vi "Pseudo_RNG.vi"() -> (3 "pseudo random value":u16)   [LabVIEW 2018]
doc: "This VI generates a sequence of pseudo random numbers using a linear feedback shift register algorithm with four taps.\n\nhttp://en.wikipedia.org/wiki/Linear_feedback_shift_register"
uses:
  <vilib>/rvi/Emulation/niFpgaSctlEmulationGetInTimedLoop.vi
  <vilib>/rvi/Emulation/niFpgaProcessEmulError.vi
  Instance           1 45Saved   Pseudo Random Number Generator (FPGA) .vi
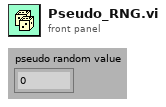
[diagram p1: front panel]
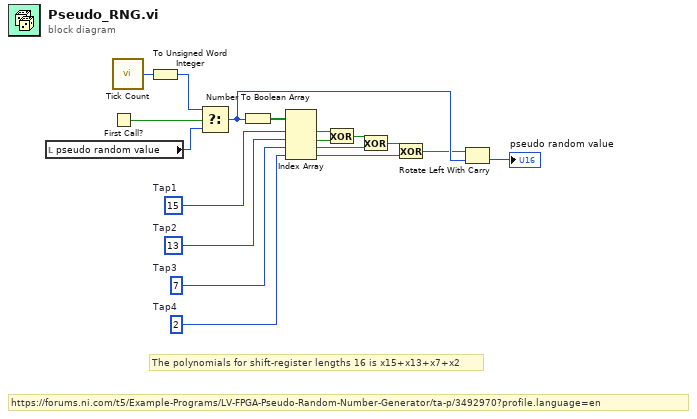
[diagram p0: block diagram]
diagram:
  w10 = 2  # Tap4
  w11 = 7  # Tap3
  w16 = 13  # Tap2
  w17 = 15  # Tap1
  # "https://forums.ni.com/t5/Example-Programs/LV-FPGA-Pseudo-Random-Number-Generator/ta-p/3492970?profile.language=en"
  # "The polynomials for shift-register lengths 16 is x15+x13+x7+x2"
  n1 = local read "pseudo random value"() -> (w9:u16)
  n2 = First Call?() -> (First Call?: T/F=w18:bool)
  n3 = call "Tick Count"() -> ("Tick Count(Ticks)"=w4:u32)
  n4 = To Unsigned Word Integer(number=w4) -> (unsigned 16bit integer=w3:u16)
  n5 = Select(t=w3, s=w18, f=w9) -> (s? t:f=w8:u16)
  n6 = Number To Boolean Array(number=w8) -> (Boolean array=w2:bool[])
  n7 = Index Array(array=w2, index #1=w17, index #2=w16, index #3=w11, index #4=w10) -> (element #1=w15:bool, element #2=w14:bool, element #3=w7:bool, element #4=w13:bool)
  n8 = Exclusive Or(1:w14, 2:w15) -> (0:w12:bool)
  n9 = Exclusive Or(1:w7, 2:w12) -> (0:w6:bool)
  n10 = Exclusive Or(1:w13, 2:w6) -> (0:w5:bool)
  n11 = Rotate Left With Carry(2:w8, 3:w5) -> (0:→"pseudo random value":u16)  [unwired: 1 out]
